vi "mclamp_auto_offset.vi"(8 "error in (no error)":errorcluster, 10 "Error in":i32, 11 "Multiclamp Handle Out":u32) -> (0 "error out":errorcluster, 3 "pipette offset (mV)":dbl)   [LabVIEW 2015]
uses:
  multiBot/patcherBot/AxMultiClampMsg.dll
panel:
  out "error out":i32
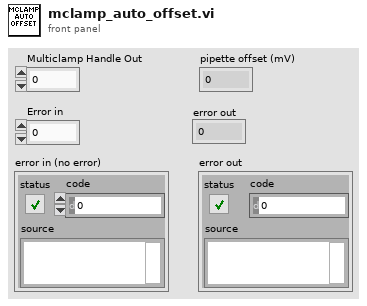
[diagram p1: front panel]
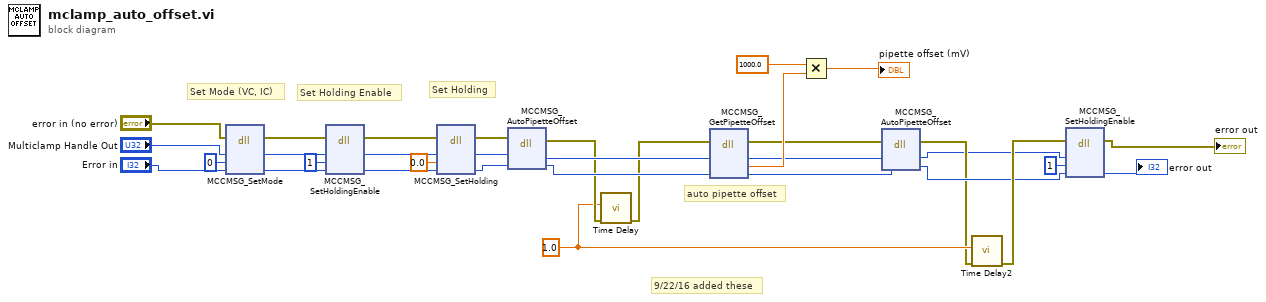
[diagram p0: block diagram]
diagram:
  w8 = 1.0 ("Delay Time (s)")
  # "9/22/16 added these"
  # "Set Holding Enable"
  # "Set Holding"
  # "Set Mode (VC, IC)"
  # "auto pipette offset"
  n1 = dll-call lib="C:/multiBot/patcherBot/AxMultiClampMsg.dll" fn="MCCMSG_SetMode"(error in="error in (no error)", "handle"="Multiclamp Handle Out", "ModeConstant"=u32 0, "error"="Error in") -> (error out=w18:errorcluster, "handle"=w16:u32, "error"=w17:i32)  [unwired: 4 in, 1 out]
  n2 = dll-call lib="C:/multiBot/patcherBot/AxMultiClampMsg.dll" fn="MCCMSG_SetHoldingEnable"(error in=w18, "handle"=w16, "ModeConstant"=1, "error"=w17) -> (error out=w19:errorcluster, "handle"=w21:u32, "error"=w20:i32)  [unwired: 4 in, 1 out]
  n3 = dll-call lib="C:/multiBot/patcherBot/AxMultiClampMsg.dll" fn="MCCMSG_SetHolding"(error in=w19, "handle"=w21, "ModeConstant"=0.0, "error"=w20) -> (error out=w26:errorcluster, "handle"=w24:u32, "error"=w25:i32)  [unwired: 4 in, 1 out]
  n4 = dll-call lib="C:/multiBot/patcherBot/AxMultiClampMsg.dll" fn="MCCMSG_AutoPipetteOffset"(error in=w26, "handle"=w24, "error"=w25) -> (error out=w10:errorcluster, "handle"=w27:u32, "error"=w28:i32)  [unwired: 3 in, 1 out]
  n5 = call "Time Delay"("error in (no error)"=w10, "Delay Time (s)"=w8) -> ("error out"=w9:errorcluster)  [unwired: 9 in]
  n6 = dll-call lib="C:/multiBot/patcherBot/AxMultiClampMsg.dll" fn="MCCMSG_GetPipetteOffset"(error in=w9, "handle"=w27, "error"=w28) -> (error out=w6:errorcluster, "handle"=w5:u32, "pdPipetteOffset"=w29:dbl, "error"=w4:i32)  [unwired: 4 in, 1 out]
  n7 = Multiply(x=1000.0, y=w29) -> (x*y=→"pipette offset (mV)":dbl)
  n8 = dll-call lib="C:/multiBot/patcherBot/AxMultiClampMsg.dll" fn="MCCMSG_AutoPipetteOffset"(error in=w6, "handle"=w5, "error"=w4) -> (error out=w2:errorcluster, "handle"=w1:u32, "error"=w3:i32)  [unwired: 3 in, 1 out]
  n9 = call "Time Delay2"("error in (no error)"=w2, "Delay Time (s)"=w8) -> ("error out"=w7:errorcluster)  [unwired: 9 in]
  n10 = dll-call lib="C:/multiBot/patcherBot/AxMultiClampMsg.dll" fn="MCCMSG_SetHoldingEnable"(error in=w7, "handle"=w1, "ModeConstant"=1, "error"=w3) -> (error out=→"error out":errorcluster, "error"=→"error out":i32)  [unwired: 5 in, 1 out]
